vi "utf_wrapper.vi"() -> (0 "Error Out":errorcluster, 3 "Application:Command Line Arguments":string[](array[string]))   [LabVIEW 2013]
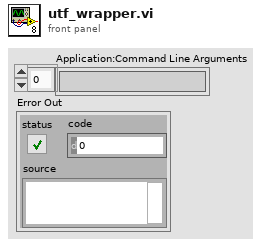
[diagram p1: front panel]
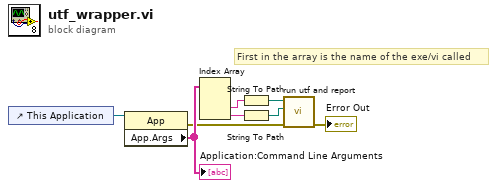
[diagram p0: block diagram]
diagram:
  # "First in the array is the name of the exe/vi called"
  n1 = control-ref of="This Application"() -> (w8:refnum<vi>)
  n2 = property class="App"(reference=w8) -> (error out=w4:errorcluster, "App.Args"=w7:string[])  [unwired: 1 in, 1 out]
  "Application:Command Line Arguments" <- w7
  n3 = Index Array(array=w7) -> (element #2=w2:string, element #3=w1:string)  [unwired: 3 in, 1 out]
  n4 = String To Path(string=w2) -> (path=w6:path)
  n5 = String To Path(string=w1) -> (path=w5:path)
  n6 = call "run utf and report.vi"("error in (no error)"=w4, "junit report file path"=w5, "project file path"=w6) -> ("Error Out"=→"Error Out":errorcluster)  [unwired: 8 in]
